vi "v0.2_dir_http.vi"(8 "error in (no error)":errorcluster, 10 "Direccion":bool, 11 "mbed.lvclass IN":refnum<class "mbed.lvclass">) -> (0 "error out":errorcluster, 3 "mbed.lvclass OUT":refnum<class "mbed.lvclass">)   [LabVIEW 2011]
doc: "<B>Dirección</B>\n\nCambiar la dirección del Servo Motor de acuerdo al valor de una variable booleana\n\n<B>dir</B> Setear la Dirección"
uses:
  C:/mbed/Transport Mechanisms/mbed/mbed.lvclass
  C:/mbed/mbed Interface/RPCFunction/RPCFunction.lvclass
panel:
  # "CAMBIA LA DIRECCIÓN DE GIRO DEL SERVOMOTOR"
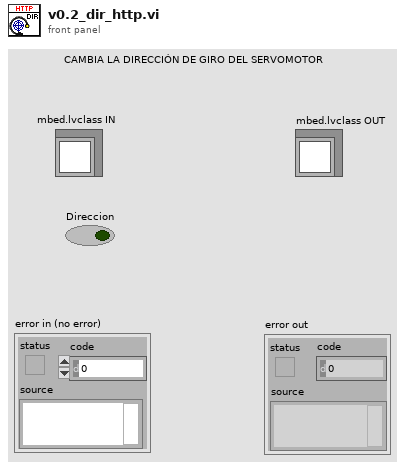
[diagram p1: front panel]
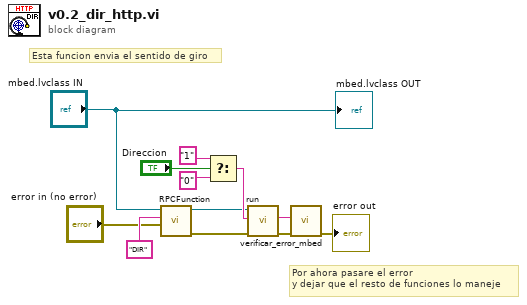
[diagram p0: block diagram]
diagram:
  # "Por ahora pasare el error\ny dejar que el resto de funciones lo maneje"
  # "Esta funcion envia el sentido de giro"
  n1 = call "RPCFunction.vi"("error in (no error)"="error in (no error)", "Existing Obj Name"="DIR", "mbed_LVLibrary.lvlib:mbed.lvclass"="mbed.lvclass IN") -> ("error out"=w6:errorcluster, "mbed_LVLibrary.lvlib:Packet.lvclass 2"=w8:refnum<class "RPCFunction.lvclass">)  [unwired: 6 in, 1 out]
  n2 = Select(t="1", s="Direccion", f="0") -> (s? t:f=w9:string)
  n3 = call "run.vi"("error in (no error)"=w6, "Input"=w9, "Packet in"=w8) -> ("error out"=w4:errorcluster, "Output"=w2:string)  [unwired: 6 in, 1 out]
  n4 = call "verificar_error_mbed.vi"("error in (no error)"=w4, "desde_mbed"=w2) -> ("error out"=→"error out":errorcluster)  [unwired: 8 in, 1 out]
  "mbed.lvclass OUT" <- "mbed.lvclass IN"
